vi "搜索一维数组函数.vi"() -> ()   [LabVIEW 2012]
panel:
  out "数组":i32[](array[numeric])
  out "元素索引":i32
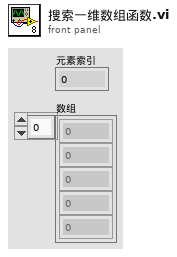
[diagram p1: front panel]
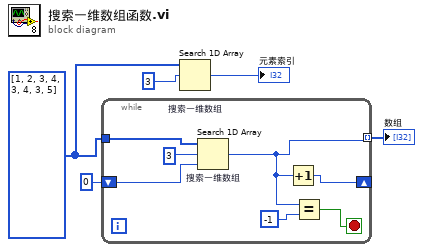
[diagram p0: block diagram]
diagram:
  w3 = i32[] [1, 2, 3, 4, 3, 4, 3, 5]
  n1 = while {
    tunnel: w3 -> [w12]
    shift-right: [w9] -> _
    shift-left: 0 -> [w10]
    tunnel: [w8] -> w1 mode=indexing
    stop <- w6 stop-if-true
    n2 = Search 1D Array "搜索一维数组"(1D array=w12, element=3 ("元素"), start index (0)=w10) -> (index of element=w8:i32)
    n3 = Increment(x=w8) -> (x+1=w9:i32)
    n4 = Equal?(x=w8, y=-1) -> (x = y?=w6:bool)
  }
  "数组" <- w1
  n5 = Search 1D Array "搜索一维数组"(1D array=w3, element=3 ("元素")) -> (index of element=→"元素索引":i32)  [unwired: 1 in]
